vi "Add Array Rows.vi"(6 "Add Button":refnum<vi>, 8 "error in (no error)":errorcluster, 9 "Element Height":u32, 10 "Number of Rows (1)":u32=1, 11 "Array":refnum<vi>) -> (0 "error out":errorcluster, 3 "Array out":refnum<vi>, 4 "Add Button out":refnum<vi>)   [LabVIEW 2017, in "UI Common.lvlib"]
uses:
  UI Common.lvlib
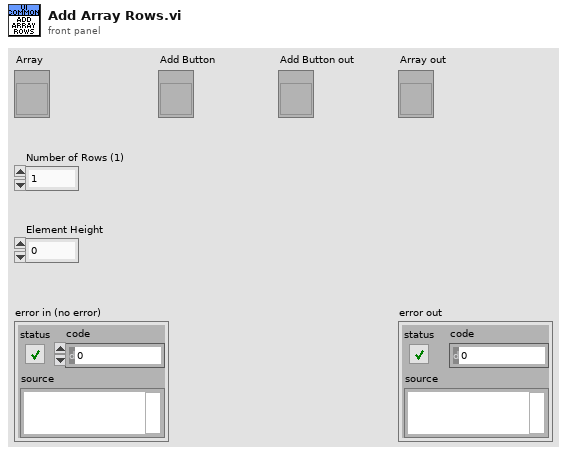
[diagram p1: front panel]
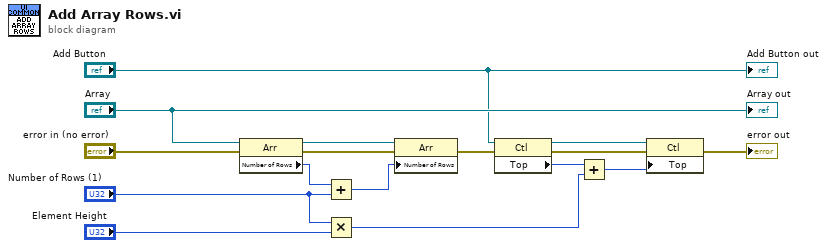
[diagram p0: block diagram]
diagram:
  n1 = property class="Arr"(reference="Array", error in="error in (no error)") -> (reference out=w14:refnum<vi>, error out=w4:errorcluster, "Number of Rows"=w15:u32)
  n2 = Add(x=w15, y="Number of Rows (1)") -> (x+y=w13:u32)
  n3 = Multiply(x="Number of Rows (1)", y="Element Height") -> (x*y=w6:u32)
  n4 = property class="Arr"(reference=w14, error in=w4, "Number of Rows"=w13) -> (error out=w3:errorcluster)  [unwired: 1 out]
  n5 = property class="Ctl"(reference="Add Button", error in=w3) -> (reference out=w12:refnum<vi>, error out=w2:errorcluster, "Top"=w11:i32)
  n6 = Add(x=w11, y=w6) -> (x+y=w10:u32)
  n7 = property class="Ctl"(reference=w12, error in=w2, "Top"=w10) -> (error out=→"error out":errorcluster)  [unwired: 1 out]
  "Array out" <- "Array"
  "Add Button out" <- "Add Button"
